vi "44-46 (SubVI).vi"(1 "String":string) -> (0 "Output":T1)   [LabVIEW 2024]
panel:
  in  "Output 2":T1
  in  "Switching Card 5":T2
  in  "Switching Card 4":T3
  in  "Switching Card 3":T4
  in  "Switching Card 2":T5
  in  "Switching Card 1":T6
  in  "Control Card":T7
  in  "Output Health Status":T8
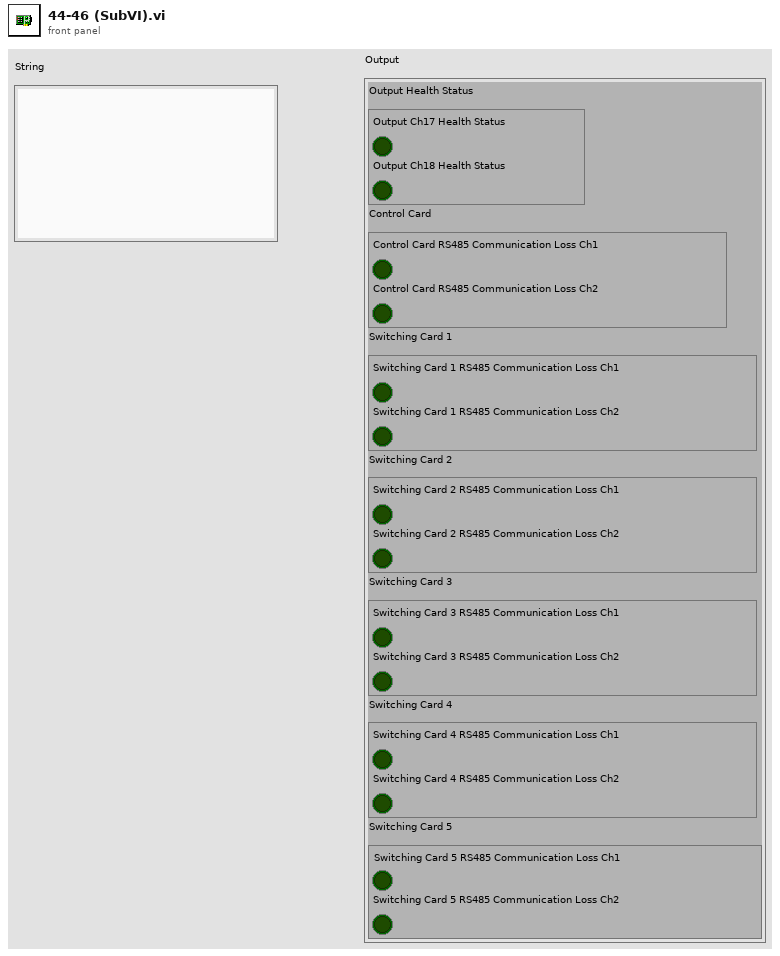
[diagram p1: front panel]
types:
  T1 = cluster{"Output Health Status":cluster{"Output Ch17 Health Status":bool, "Output Ch18 Health Status":bool}, "Control Card":cluster{"Control Card RS485 Communication Loss Ch1":bool, "Control Card RS485 Communication Loss Ch2":bool}, "Switching Card 1":cluster{"Switching Card 1 RS485 Communication Loss Ch1":bool, "Switching Card 1 RS485 Communication Loss Ch2":bool}, "Switching Card 2":cluster{"Switching Card 2 RS485 Communication Loss Ch1":bool, "Switching Card 2 RS485 Communication Loss Ch2":bool}, "Switching Card 3":cluster{"Switching Card 3 RS485 Communication Loss Ch1":bool, "Switching Card 3 RS485 Communication Loss Ch2":bool}, "Switching Card 4":cluster{"Switching Card 4 RS485 Communication Loss Ch1":bool, "Switching Card 4 RS485 Communication Loss Ch2":bool}, "Switching Card 5":cluster{"Switching Card 5 RS485 Communication Loss Ch1":bool, "Switching Card 5 RS485 Communication Loss Ch2":bool}}
  T2 = cluster{"Switching Card 5 RS485 Communication Loss Ch1":bool, "Switching Card 5 RS485 Communication Loss Ch2":bool}
  T3 = cluster{"Switching Card 4 RS485 Communication Loss Ch1":bool, "Switching Card 4 RS485 Communication Loss Ch2":bool}
  T4 = cluster{"Switching Card 3 RS485 Communication Loss Ch1":bool, "Switching Card 3 RS485 Communication Loss Ch2":bool}
  T5 = cluster{"Switching Card 2 RS485 Communication Loss Ch1":bool, "Switching Card 2 RS485 Communication Loss Ch2":bool}
  T6 = cluster{"Switching Card 1 RS485 Communication Loss Ch1":bool, "Switching Card 1 RS485 Communication Loss Ch2":bool}
  T7 = cluster{"Control Card RS485 Communication Loss Ch1":bool, "Control Card RS485 Communication Loss Ch2":bool}
  T8 = cluster{"Output Ch17 Health Status":bool, "Output Ch18 Health Status":bool}
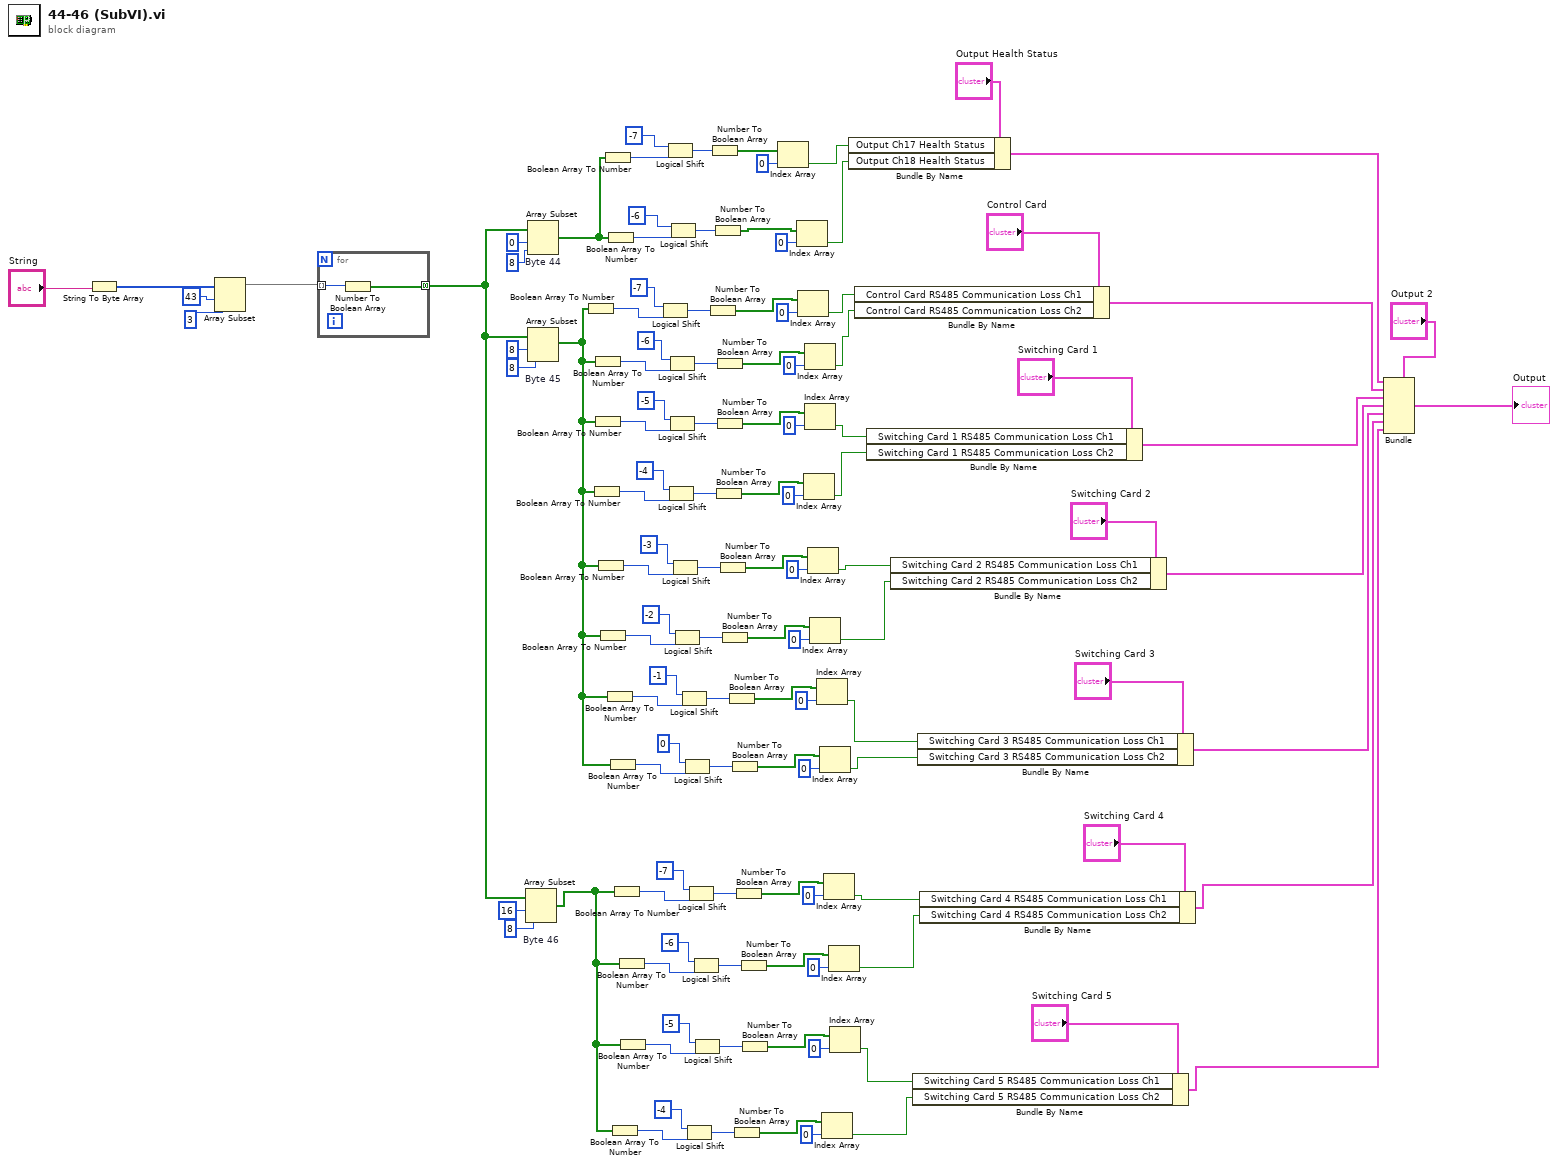
[diagram p0: block diagram]
diagram:
  n1 = String To Byte Array(string="String") -> (unsigned byte array=w107:u8[])
  n2 = Array Subset(array=w107, index=43, length=3) -> (w104:u8[])
  n3 = for {
    tunnel: w104 -> [w117] mode=indexing
    tunnel: [w116] -> w114 mode=concatenating
    n4 = Number To Boolean Array(number=w117) -> (Boolean array=w116:bool[])
  }
  n5 = Array Subset "Byte 46"(array=w114, index=16, length=8) -> (w31:bool[])
  n6 = Array Subset "Byte 44"(array=w114, index=0, length=8) -> (w97:bool[])
  n7 = Array Subset "Byte 45"(array=w114, index=8, length=8) -> (w52:bool[])
  n8 = Boolean Array To Number(Boolean array=w52) -> (number=w92:u32)
  n9 = Boolean Array To Number(Boolean array=w52) -> (number=w73:u32)
  n10 = Boolean Array To Number(Boolean array=w52) -> (number=w83:u32)
  n11 = Boolean Array To Number(Boolean array=w52) -> (number=w82:u32)
  n12 = Boolean Array To Number(Boolean array=w52) -> (number=w72:u32)
  n13 = Boolean Array To Number(Boolean array=w52) -> (number=w63:u32)
  n14 = Boolean Array To Number(Boolean array=w97) -> (number=w98:u32)
  n15 = Boolean Array To Number(Boolean array=w52) -> (number=w62:u32)
  n16 = Boolean Array To Number(Boolean array=w97) -> (number=w103:u32)
  n17 = Boolean Array To Number(Boolean array=w52) -> (number=w53:u32)
  n18 = Boolean Array To Number(Boolean array=w31) -> (number=w32:u32)
  n19 = Boolean Array To Number(Boolean array=w31) -> (number=w51:u32)
  n20 = Boolean Array To Number(Boolean array=w31) -> (number=w42:u32)
  n21 = Boolean Array To Number(Boolean array=w31) -> (number=w41:u32)
  n22 = Logical Shift(y=i16 -7, x=w92) -> (x << y=w90:u32)
  n23 = Logical Shift(y=i16 -7, x=w98) -> (x << y=w100:u32)
  n24 = Logical Shift(y=i16 -4, x=w73) -> (x << y=w74:u32)
  n25 = Logical Shift(y=i16 -6, x=w83) -> (x << y=w85:u32)
  n26 = Logical Shift(y=i16 -5, x=w82) -> (x << y=w81:u32)
  n27 = Logical Shift(y=i16 -6, x=w103) -> (x << y=w101:u32)
  n28 = Logical Shift(y=i16 -3, x=w72) -> (x << y=w71:u32)
  n29 = Logical Shift(y=i16 -2, x=w63) -> (x << y=w64:u32)
  n30 = Logical Shift(y=i16 -1, x=w62) -> (x << y=w61:u32)
  n31 = Logical Shift(y=i16 0, x=w53) -> (x << y=w54:u32)
  n32 = Logical Shift(y=i16 -4, x=w32) -> (x << y=w33:u32)
  n33 = Logical Shift(y=i16 -7, x=w51) -> (x << y=w50:u32)
  n34 = Logical Shift(y=i16 -6, x=w42) -> (x << y=w43:u32)
  n35 = Logical Shift(y=i16 -5, x=w41) -> (x << y=w40:u32)
  n36 = Number To Boolean Array(number=w90) -> (Boolean array=w88:bool[])
  n37 = Number To Boolean Array(number=w100) -> (Boolean array=w96:bool[])
  n38 = Number To Boolean Array(number=w101) -> (Boolean array=w93:bool[])
  n39 = Number To Boolean Array(number=w74) -> (Boolean array=w76:bool[])
  n40 = Number To Boolean Array(number=w85) -> (Boolean array=w87:bool[])
  n41 = Number To Boolean Array(number=w81) -> (Boolean array=w79:bool[])
  n42 = Number To Boolean Array(number=w71) -> (Boolean array=w69:bool[])
  n43 = Number To Boolean Array(number=w64) -> (Boolean array=w66:bool[])
  n44 = Number To Boolean Array(number=w61) -> (Boolean array=w59:bool[])
  n45 = Number To Boolean Array(number=w54) -> (Boolean array=w56:bool[])
  n46 = Number To Boolean Array(number=w33) -> (Boolean array=w35:bool[])
  n47 = Number To Boolean Array(number=w50) -> (Boolean array=w48:bool[])
  n48 = Number To Boolean Array(number=w43) -> (Boolean array=w45:bool[])
  n49 = Number To Boolean Array(number=w40) -> (Boolean array=w38:bool[])
  n50 = Index Array(array=w96, index=0) -> (element=w30:bool)
  n51 = Index Array(array=w93, index=0) -> (element=w29:bool)
  n52 = Index Array(array=w88, index=0) -> (element=w28:bool)
  n53 = Index Array(array=w76, index=0) -> (element=w25:bool)
  n54 = Index Array(array=w87, index=0) -> (element=w27:bool)
  n55 = Index Array(array=w79, index=0) -> (element=w26:bool)
  n56 = Index Array(array=w69, index=0) -> (element=w24:bool)
  n57 = Index Array(array=w66, index=0) -> (element=w23:bool)
  n58 = Index Array(array=w59, index=0) -> (element=w22:bool)
  n59 = Index Array(array=w56, index=0) -> (element=w21:bool)
  n60 = Index Array(array=w35, index=0) -> (element=w17:bool)
  n61 = Index Array(array=w48, index=0) -> (element=w20:bool)
  n62 = Index Array(array=w45, index=0) -> (element=w19:bool)
  n63 = Index Array(array=w38, index=0) -> (element=w18:bool)
  n64 = Bundle By Name(cluster="Output Health Status", "Output Ch17 Health Status"=w30, "Output Ch18 Health Status"=w29) -> (w8:T8)
  n65 = Bundle By Name(cluster="Control Card", "Control Card RS485 Communication Loss Ch1"=w28, "Control Card RS485 Communication Loss Ch2"=w27) -> (w7:T7)
  n66 = Bundle By Name(cluster="Switching Card 1", "Switching Card 1 RS485 Communication Loss Ch1"=w26, "Switching Card 1 RS485 Communication Loss Ch2"=w25) -> (w6:T6)
  n67 = Bundle By Name(cluster="Switching Card 2", "Switching Card 2 RS485 Communication Loss Ch1"=w24, "Switching Card 2 RS485 Communication Loss Ch2"=w23) -> (w5:T5)
  n68 = Bundle By Name(cluster="Switching Card 5", "Switching Card 5 RS485 Communication Loss Ch1"=w18, "Switching Card 5 RS485 Communication Loss Ch2"=w17) -> (w2:T2)
  n69 = Bundle By Name(cluster="Switching Card 3", "Switching Card 3 RS485 Communication Loss Ch1"=w22, "Switching Card 3 RS485 Communication Loss Ch2"=w21) -> (w4:T4)
  n70 = Bundle By Name(cluster="Switching Card 4", "Switching Card 4 RS485 Communication Loss Ch1"=w20, "Switching Card 4 RS485 Communication Loss Ch2"=w19) -> (w3:T3)
  n71 = Bundle(cluster="Output 2", "Output Health Status"=w8, "Control Card"=w7, "Switching Card 1"=w6, "Switching Card 2"=w5, "Switching Card 3"=w4, "Switching Card 4"=w3, "Switching Card 5"=w2) -> (→"Output":T1)
